vi "NEagle Tester.vi"() -> ()   [LabVIEW 2015]
panel:
  out "appended array":bool[][](array[boolean])
  in  "stop":bool
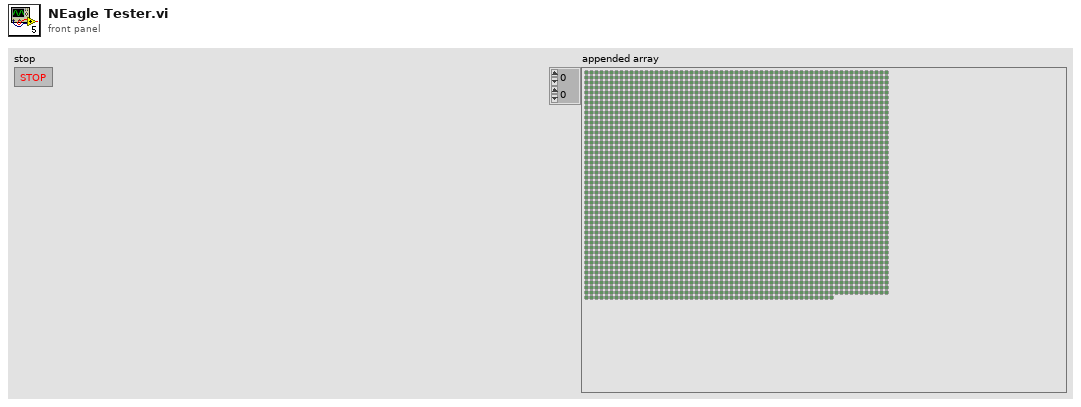
[diagram p1: front panel]
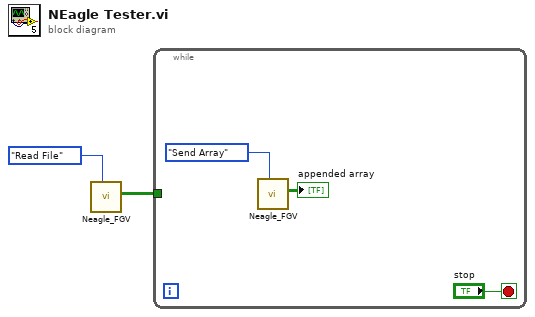
[diagram p0: block diagram]
diagram:
  n1 = call "Neagle_FGV.vi"("Options"=enum16{"Read File", "Send Array"}."Read File") -> ("appended array"=w1:bool[][])  [unwired: 10 in]
  n2 = while {
    tunnel: w1 -> [_]
    stop <- "stop" stop-if-true
    n3 = call "Neagle_FGV.vi"("Options"=enum16{"Read File", "Send Array"}."Send Array") -> ("appended array"=→"appended array":bool[][])  [unwired: 10 in]
  }
